vi "test_ImageAssemblerDL090211Frame.vi"() -> ()   [LabVIEW 2010, in "ImageAssemblerDL090211Frame.lvclass"]
uses:
  ImageAssemblerDL090211Frame.lvclass
  main/labview_source/type_definitions/clusters/controls_refs.ctl
  GenericImageAssembler/GenericImageAssembler/trigger_enum.ctl
  common/classes/Image/Image/Image.lvclass
  ImageAssemblerDL090211Scaffold/ImageAssemblerDL090211Scaffold/ImageAssemblerDL090211Scaffold.lvclass
  GenericImageAssembler/GenericImageAssembler/GenericImageAssembler.lvclass
panel:
  out "event loop counter":i32
  in  "start":bool
  in  "image path":path
  in  "insert":bool
  in  "number of pixels to insert":i32=8000
  in  "stop":bool
  in  "create button":bool
  in  "number of channels":i32=1 min=1 max=4
  in  "x resolution":i32=256
  in  "y resolution":i32=256
  in  "repetitions":i32=3
  # "Test VI for ImageAssemblerDL090211Frame"
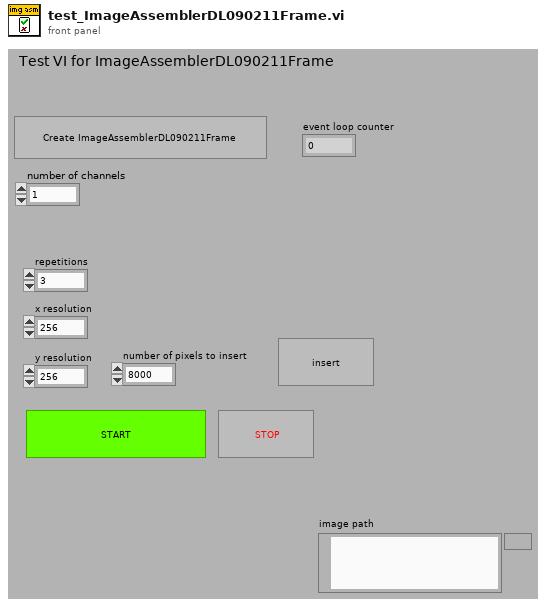
[diagram p1: front panel]
types:
  T1 = typedef "controls_refs.ctl" = cluster{"scan start button":refnum<vi>, "tabs":cluster{"main":refnum<vi>, "settings":refnum<vi>}, "subpanels":cluster{"imagingMode":refnum<vi>, "scanHead":refnum<vi>, "display":refnum<vi>, "experimentController":refnum<vi>, "instrument":refnum<vi>, "stage":refnum<vi>, "stimulator":refnum<vi>, "dataCollection":refnum<vi>, "analyser":refnum<vi>, "daq":refnum<vi>, "imageAssembler":refnum<vi>}, "drop-downs":cluster{"run mode":refnum<vi>, "imagingMode":refnum<vi>, "experimentalController":refnum<vi>, "objective":refnum<vi>}, "status lights":cluster{"experimentController":refnum<vi>, "imagingMode":refnum<vi>, "scanHead":refnum<vi>, "daq":refnum<vi>, "imageAssembler":refnum<vi>, "dataCollection":refnum<vi>, "display":refnum<vi>, "analyser":refnum<vi>, "stage":refnum<vi>, "stimulator":refnum<vi>, "instrument":refnum<vi>}, "message":refnum<vi>, "stimulator enabled?":refnum<vi>, "saving":cluster{"data folder path":refnum<vi>, "file base name":refnum<vi>, "notebook":refnum<vi>}, "progress bar":refnum<vi>, "update icon":refnum<vi>, "title":refnum<vi>, "main vi":refnum<vi>, "user":refnum<vi>, "exit_button":refnum<vi>, "CPU usage %":refnum<vi>}
  T2 = typedef "GenericImageAssembler.lvclass/trigger_enum.ctl" = enum16{"NULL", "start", "stop"}
  T3 = typedef "plugin_specification.ctl" = cluster{"class path":string, "configuration":string, "label":string, "settings name":string}
  T4 = typedef "XComponentSpecification.xctl/data.ctl" = cluster{"class path":string, "configuration":string, "label":string, "settings name":string}
  T5 = typedef "Image Type" = u32
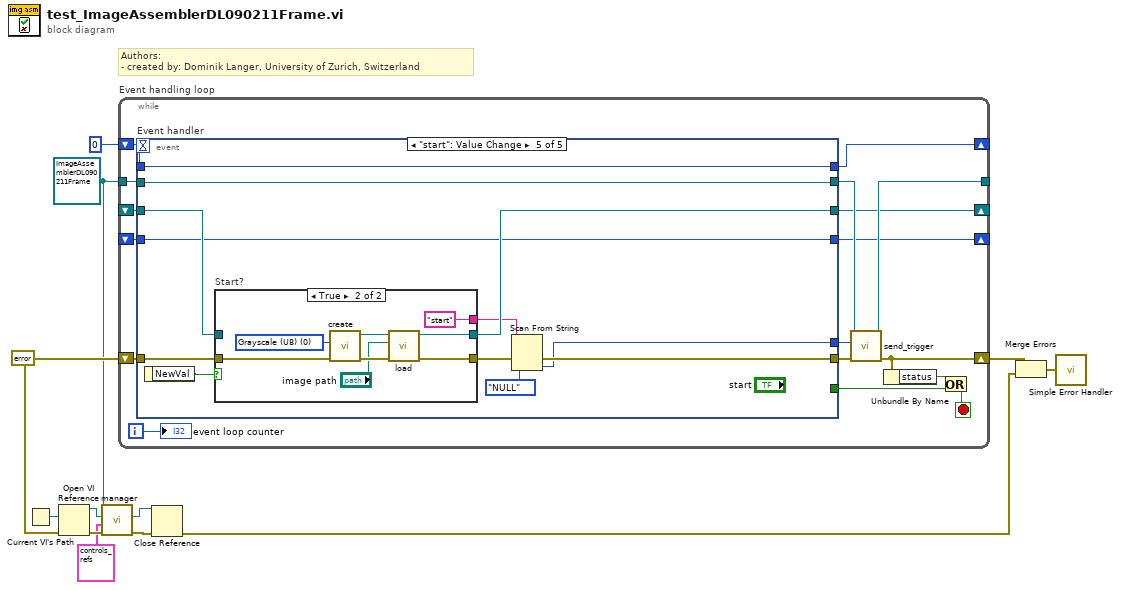
[diagram p0: block diagram]
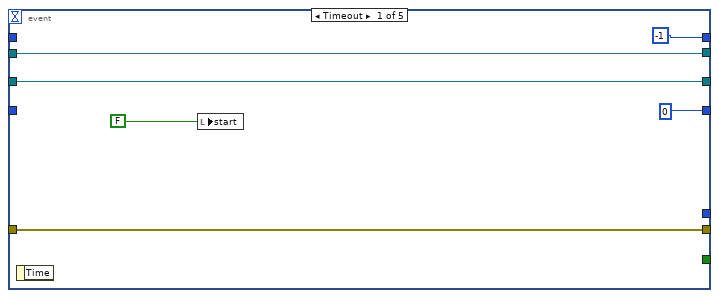
[diagram p2: hidden frame]
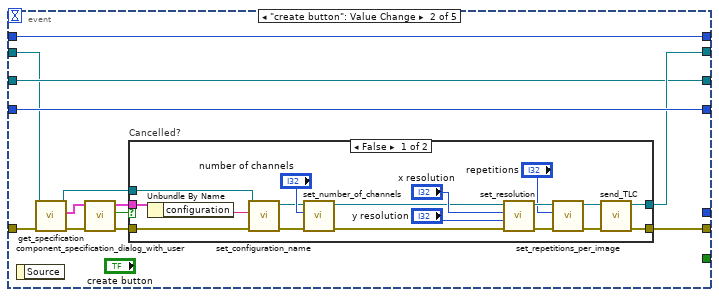
[diagram p3: hidden frame]
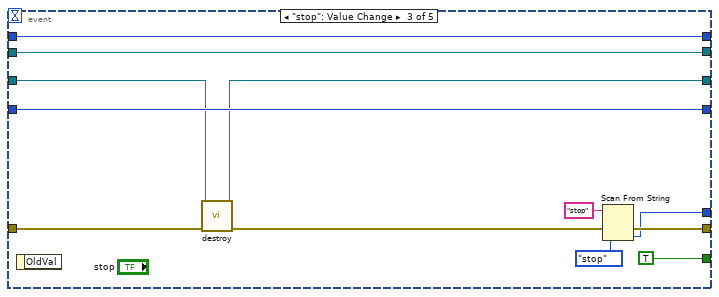
[diagram p5: hidden frame]
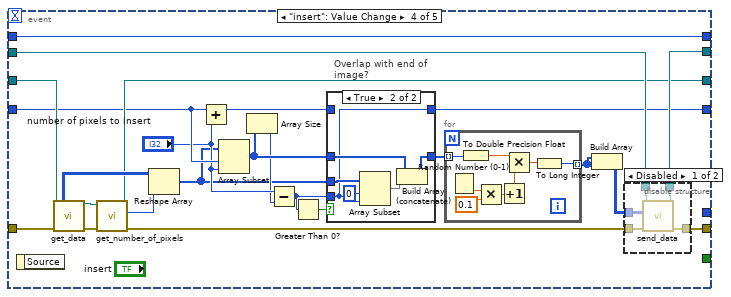
[diagram p6: hidden frame]
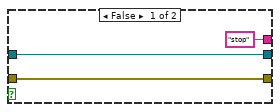
[diagram p9: hidden frame]
diagram:
  w6 = refnum<class "ImageAssemblerDL090211Frame.lvclass"> refnum ("ImageAssemblerDL090211Frame.lvclass")
  w11 = errorcluster {"status"=FALSE, "code"=0, "source"=""} ("error out")
  # "Authors: \n- created by: Dominik Langer, University of Zurich, Switzerland"
  n1 = Current VI's Path() -> (path=w7:path)
  n2 = Open VI Reference(vi path=w7, error in (no error)=w11) -> (vi reference=w1:refnum<vi>, error out=w5:errorcluster)  [unwired: 4 in]
  n3 = call-dynamic "manager.vi"("error in (no error)"=w5, "control references"=T1 {"scan start button"=refnum, "tabs"={"main"=refnum, "settings"=refnum}, "subpanels"={"imagingMode"=refnum, "scanHead"=refnum, "display"=refnum, "experimentController"=refnum, "instrument"=refnum, "stage"=refnum, "stimulator"=refnum, "dataCollection"=refnum, "analyser"=refnum, "daq"=refnum, "imageAssembler"=refnum}, "drop-downs"={"run mode"=refnum, "imagingMode"=refnum, "experimentalController"=refnum, "objective"=refnum}, "status lights"={"experimentController"=refnum, "imagingMode"=refnum, "scanHead"=refnum, "daq"=refnum, "imageAssembler"=refnum, "dataCollection"=refnum, "display"=refnum, "analyser"=refnum, "stage"=refnum, "stimulator"=refnum, "instrument"=refnum}, "message"=refnum, "stimulator enabled?"=refnum, "saving"={"data folder path"=refnum, "file base name"=refnum, "notebook"=refnum}, "progress bar"=refnum, "update icon"=refnum, "title"=refnum, "main vi"=refnum, "user"=refnum, "exit_button"=refnum, "CPU usage %"=refnum}, "top-level VI ref in"=w1, "GenericToplevelComponent in"=w6) -> ("error out"=w3:errorcluster, "top-level VI ref out"=w4:refnum<vi>)  [unwired: 5 in, 1 out]
  n4 = while "Event handling loop" {
    shift-right: [w28] -> _
    shift-left: 0 -> [w29]
    shift-right: [w17] -> w10
    shift-left: w11 -> [w27]
    shift-right: [w20] -> _
    shift-left: _ -> [w21]
    shift-right: [w19] -> _
    shift-left: _ -> [w18]
    tunnel: w6 -> [w24]
    tunnel: [w22] -> _
    i -> [w13]
    stop <- w14 stop-if-true
    n5 = event "Event handler" shown="[4] \"start\": Value Change" {
      selector: _ -> [_ _ _ _ _]
      dyn-events: _ -> [_ _ _ _ _]
      timeout: w29 -> [_ _ _ _ _]
      tunnel: [-1 w48 w80 w104 w137] -> w28
      tunnel: w29 -> [_ w48 w80 w104 w137]
      tunnel: [w30 w46 w71 w103 w128] -> w26
      tunnel: w27 -> [w30 w42 w76 w100 w135]
      tunnel: [_ _ w70 _ w126] -> w25
      tunnel: [_ _ TRUE _ _] -> w16
      tunnel: w24 -> [w32 w39 w78 w102 w136]
      tunnel: [w32 w45 w78 w101 w136] -> w23
      tunnel: w21 -> [w31 w44 w75 w99 w133]
      tunnel: [w31 w44 w74 w94 w132] -> w20
      tunnel: [0 w47 w77 w84 w131] -> w19
      tunnel: w18 -> [_ w47 w77 w92 w131]
      event Timeout {
        n6 = event-data() -> ()  [unwired: 2 out]
        n7 = local write "start"(FALSE) -> ()
      }
      event "create button": Value Change {
        n8 = event-data() -> ()  [unwired: 2 out]
        n9 = call-dynamic "get_specification.vi"("error in (no error)"=w42, "GenericPlugin in"=w39) -> ("error out"=w41:errorcluster, "component specification"=w40:T3, "GenericPlugin out"=w38:refnum<class "ImageAssemblerDL090211Frame.lvclass">)  [unwired: 6 in, 1 out]
        n10 = call "component_specification_dialog_with_user.vi"("error in (no error)"=w41, "component specification in"=w40) -> ("error out"=w43:errorcluster, "cancelled?"=w36:bool, "component specification out"=w37:T4)  [unwired: 7 in]
        n11 = case "Cancelled?" shown="False" w36 {
          tunnel: [w59 w68] -> w46
          tunnel: [w55 w67] -> w45
          tunnel: w43 -> [w52 w68]
          tunnel: w38 -> [w51 w67]
          tunnel: w37 -> [w50 _]
          frame False {
            n12 = Unbundle By Name(w50) -> ("configuration"=w49:string)
            n13 = call-dynamic "set_configuration_name.vi"("error in (no error)"=w52, "configuration"=w49, "GenericPlugin.lvclass in"=w51) -> ("error out"=w53:errorcluster, "GenericPlugin.lvclass out"=w54:refnum<class "ImageAssemblerDL090211Frame.lvclass">)  [unwired: 7 in]
            n14 = call-dynamic "set_number_of_channels.vi"("error in (no error)"=w53, "number of channels"="number of channels", "GenericImageAssembler.lvclass in"=w54) -> ("error out"=w60:errorcluster, "GenericImageAssembler.lvclass out"=w56:refnum<class "ImageAssemblerDL090211Frame.lvclass">)  [unwired: 7 out]
            n15 = call "set_resolution.vi"("error in (no error)"=w60, "y resolution"="y resolution", "x resolution"="x resolution", "DL090211FrameImageAssembler.lvclass in"=w56) -> ("error out"=w58:errorcluster, "DL090211FrameImageAssembler.lvclass out"=w63:refnum<class "ImageAssemblerDL090211Frame.lvclass">)  [unwired: 6 out]
            n16 = call "set_repetitions_per_image.vi"("error in (no error)"=w58, "repetitions per image"="repetitions", "DL090211ImageAssemblerScaffold.lvclass in"=w63) -> ("error out"=w57:errorcluster, "DL090211ImageAssemblerScaffold.lvclass out"=w61:refnum<class "ImageAssemblerDL090211Frame.lvclass">)  [unwired: 7 out]
            n17 = call-dynamic "send_TLC.vi"("error in (no error)"=w57, "GenericToplevelComponent in"=w61) -> ("error out"=w59:errorcluster, "GenericToplevelComponent out"=w55:refnum<class "ImageAssemblerDL090211Frame.lvclass">)  [unwired: 8 in]
          }
          frame True {
          }
        }
      }
      event "stop": Value Change {
        n18 = event-data() -> ()  [unwired: 2 out]
        n19 = call-dynamic "destroy.vi"("error in (no error)"=w76, "Image in"=w75) -> ("error out"=w72:errorcluster, "Image out"=w74:refnum<class "Image.lvclass">)  [unwired: 8 in]
        n20 = Scan From String(input string="stop", error in=w72, default 1=trigger_enum."stop" ("Enum")) -> (error out=w71:errorcluster, output 1=w70:T2)  [unwired: 2 in, 2 out]
      }
      event "insert": Value Change {
        n21 = event-data() -> ()  [unwired: 2 out]
        n22 = call-dynamic "get_data.vi"("Image in"=w99, "error in (no error)"=w100) -> ("Image Pixels (U8)"=w98:u8[][], "Image out"=w95:refnum<class "Image.lvclass">, "error out"=w97:errorcluster)  [unwired: 11 out]
        n23 = call "get_number_of_pixels.vi"("error in (no error)"=w97, "Image in"=w95) -> ("error out"=w96:errorcluster, "number of pixels"=w93:i32, "Image out"=w94:refnum<class "Image.lvclass">)  [unwired: 7 out]
        n24 = Reshape Array(w98, w93) -> (w86:u8[])
        n25 = Add(x=w92, y="number of pixels to insert") -> (x+y=w85:i32)
        n26 = Array Subset(array=w86, index=w92, length="number of pixels to insert") -> (w91:u8[])
        n27 = Array Size(array=w91) -> (size(s)=w89:i32)
        n28 = Subtract(x="number of pixels to insert", y=w89) -> (x-y=w87:i32)
        n29 = Greater Than 0?(x=w87) -> (x > 0?=w88:bool)
        n30 = case "Overlap with end of image?" shown="True" w88 {
          tunnel: w91 -> [w119 w121]
          tunnel: [w119 w123] -> w83
          tunnel: w87 -> [_ w120]
          tunnel: w86 -> [_ w122]
          tunnel: [w118 w120] -> w84
          tunnel: w85 -> [w118 _]
          frame False {
          }
          frame True {
            n31 = Array Subset(array=w122, index=0, length=w120) -> (w124:u8[])
            n32 = Build Array (concatenate)(w121, w124) -> (w123:u8[])
          }
        }
        n33 = for {
          tunnel: w83 -> [w112] mode=indexing
          tunnel: [w111] -> w82 mode=indexing
          n34 = Random Number (0-1)() -> (number: 0 to 1=w115:dbl)
          n35 = To Double Precision Float(number=w112) -> (double precision float=w116:dbl)
          n36 = Multiply(x=w115, y=0.1) -> (x*y=w114:dbl)
          n37 = Increment(x=w114) -> (x+1=w113:dbl)
          n38 = Multiply(x=w116, y=w113) -> (x*y=w117:dbl)
          n39 = To Long Integer(number=w117) -> (32bit integer=w111:i32)
        }
        n40 = Build Array(w82, w82) -> (w81:i32[][])
        n41 = disable-structure shown="Disabled" {
          disable-tunnel: [w108 _] -> w103
          disable-tunnel: w102 -> [w107 _]
          disable-tunnel: [w106 _] -> w101
          disable-tunnel: w96 -> [w109 _]
          disable-tunnel: w81 -> [w105 _]
          frame Disabled {
            n42 = call-dynamic "send_data.vi"("error in (no error)"=w109, "data"=w105, "GenericToplevelComponent in"=w107) -> ("error out"=w108:errorcluster, "GenericToplevelComponent out"=w106:refnum<class "ImageAssemblerDL090211Frame.lvclass">)  [unwired: 6 in, 1 out]
          }
          frame Enabled {
          }
        }
      }
      event "start": Value Change {
        n43 = event-data() -> ("NewVal"=w134:bool)  [unwired: 1 out]
        n44 = case "Start?" shown="True" w134 {
          tunnel: w135 -> [w140 w148]
          tunnel: [w140 w145] -> w129
          tunnel: [w139 w142] -> w132
          tunnel: w133 -> [w139 _]
          tunnel: ["stop" "start"] -> w127
          frame False {
          }
          frame True {
            w147 = T5 0 items=["Grayscale (U8)", "Grayscale (I16)", "Grayscale (SGL)", "Complex (CSG)", "RGB (U32)", "HSL (U32)", "RGB (U64)", "Grayscale (U16)"] ("Image Type")
            n45 = call "create.vi"("error in (no error)"=w148, "Image Type"=w147) -> ("error out"=w146:errorcluster, "Image out"=w144:refnum<class "Image.lvclass">)  [unwired: 2 in, 6 out]
            n46 = call-dynamic "load.vi"("error in (no error)"=w146, "Path"="image path", "Image in"=w144) -> ("error out"=w145:errorcluster, "Image out"=w142:refnum<class "Image.lvclass">)  [unwired: 1 in, 6 out]
          }
        }
        n47 = Scan From String(input string=w127, error in=w129, default 1=trigger_enum."NULL" ("Enum")) -> (error out=w128:errorcluster, output 1=w126:T2)  [unwired: 2 in, 2 out]
      }
    }
    n48 = call-dynamic "send_trigger.vi"("error in (no error)"=w26, "trigger"=w25, "GenericImageAssembler in"=w23) -> ("error out"=w17:errorcluster, "GenericImageAssembler out"=w22:refnum<class "ImageAssemblerDL090211Frame.lvclass">)  [unwired: 7 out]
    n49 = Unbundle By Name(w17) -> ("status"=w15:bool)
    n50 = Or(x=w15, y=w16) -> (x .or. y?=w14:bool)
    "event loop counter" <- w13
  }
  n51 = Close Reference(reference=w4, error in (no error)=w3) -> (error out=w9:errorcluster)
  n52 = Merge Errors(w10, w9) -> (w8:errorcluster)
  n53 = call <vilib>:"Simple Error Handler.vi"("error in (no error)"=w8) -> ()  [unwired: 4 in, 5 out]
